vi "Set Point.vi"(8 "error in (no error)":errorcluster, 10 "Set point":dbl, 11 "Arduino Temperature Controller Driver in":refnum<class "Arduino Temperature Controller Driver.lvclass">) -> (0 "error out":errorcluster, 3 "Arduino Temperature Controller Driver out":refnum<class "Arduino Temperature Controller Driver.lvclass">)   [LabVIEW 2018, in "Arduino Temperature Controller Driver.lvclass"]
uses:
  Arduino Temperature Controller Driver.lvclass
  C:/github/NHMFL_Core/Libraries/Instruments/VISA Instrument/VISA Instrument.lvclass
  VISA Instrument/VISA Instrument.lvclass/VISA Instrument.ctl
  VISA Instrument/Read VISA resource.vi
  VISA Instrument/Write VISA resource.vi
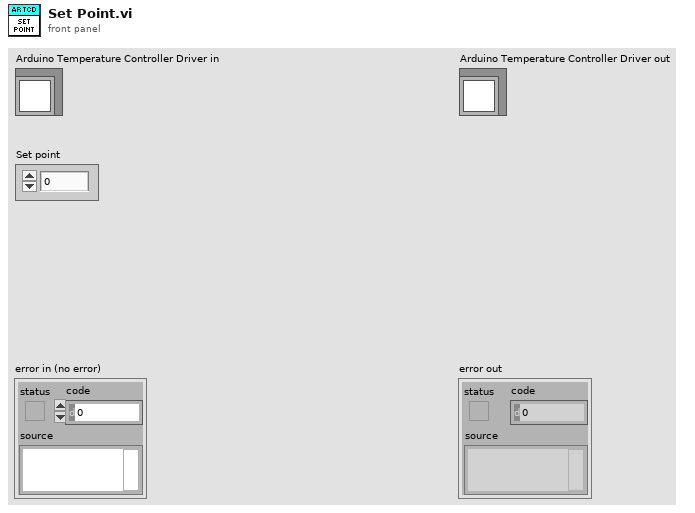
[diagram p1: front panel]
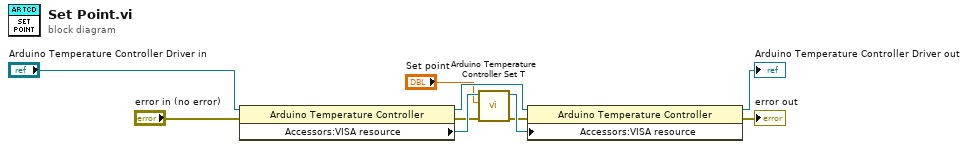
[diagram p0: block diagram]
diagram:
  n1 = property class="Arduino Temperature Controller "(reference="Arduino Temperature Controller Driver in", error in="error in (no error)") -> (reference out=w6:refnum<class "Arduino Temperature Controller Driver.lvclass">, error out=w7:errorcluster, "Accessors:VISA resource"=w9:refnum<visa-resource-name>)
  n2 = call "Arduino Temperature Controller Set T.vi"("Error In"=w7, "Set point"="Set point", "VISA resource name"=w9) -> ("Error Out"=w5:errorcluster, "VISA resource name out"=w8:refnum<visa-resource-name>)  [unwired: 7 in]
  n3 = property class="Arduino Temperature Controller "(reference=w6, error in=w5, "Accessors:VISA resource"=w8) -> (reference out=→"Arduino Temperature Controller Driver out":refnum<class "Arduino Temperature Controller Driver.lvclass">, error out=→"error out":errorcluster)
